vi "ConfigDlg.vi"(8 "error in (no error)":errorcluster, 11 "NiPxi6733 in":refnum<class "NiPxi6733.lvclass">) -> (0 "error out":errorcluster, 2 "Changed":bool, 3 "NiPxi6733 out":refnum<class "NiPxi6733.lvclass">)   [LabVIEW 2014, in "FgenPlugins.lvlib" / "NiPxi6733.lvclass"]
uses:
  NiPxi6733.lvclass
  TypeDefs/Channels.ctl
  TypeDefs/Channel.ctl
  TypeDefs/RefClk.ctl
  TypeDefs/clTriggers.ctl
  TypeDefs/Trigger.ctl
  TypeDefs/TriggerType.ctl
  Typedefs/Timebase.ctl
  FgenPluginBaseClass/FgenPluginsBase.lvclass/FgenPluginsBase.ctl
  NiPxi6733.lvclass/NiPxi6733.ctl
  <userlib>/NIST/BaseClasses/BasePlugin_class/BasePlugin.lvclass/BasePlugin.ctl
  <userlib>/NIST/BaseClasses/BasePlugin_class/Accessors/Read PluginIniFilePath.vi
  FgenPluginBaseClass/Accessors/Write reference clock source (Internal).vi
  Accessors/Write SampleRate.vi
  FgenPluginBaseClass/Accessors/Write Triggers.vi
  Accessors/Write Timebase.vi
  FgenPluginBaseClass/Accessors/Write Channels.vi
  FgenPluginBaseClass/Accessors/Read FunctionClass.vi
  Accessors/Read SampleRate.vi
  FgenPluginBaseClass/Accessors/Write FunctionClass.vi
  FgenPluginBaseClass/Accessors/Read Channels.vi
  FgenPluginBaseClass/Accessors/Read reference clock source (Internal).vi
  FgenPluginBaseClass/Read Triggers.vi
  Accessors/Read Timebase.vi
  MemberClasses/FunctionBaseClass/FunctionBase.lvclass
  <vilib>/Utility/config.llb/NI_LVConfig.lvlib
  FgenPlugins.lvlib
panel:
  in  "Timebase":T1={"source"="/PXI1Slot6/PXI_Trig1", "rate"=18000000.0}
  in  "Triggers":T2
  in  "SampleRate":dbl
  in  "btnDone":bool
  in  "btnCancel":bool
  in  "btnFuncConfig":bool
  in  "RefClk":T5 caption="reference clock source" items=["Internal"=0, "External"=1, "RTSI Clock"=101]
  in  "Channels":T6
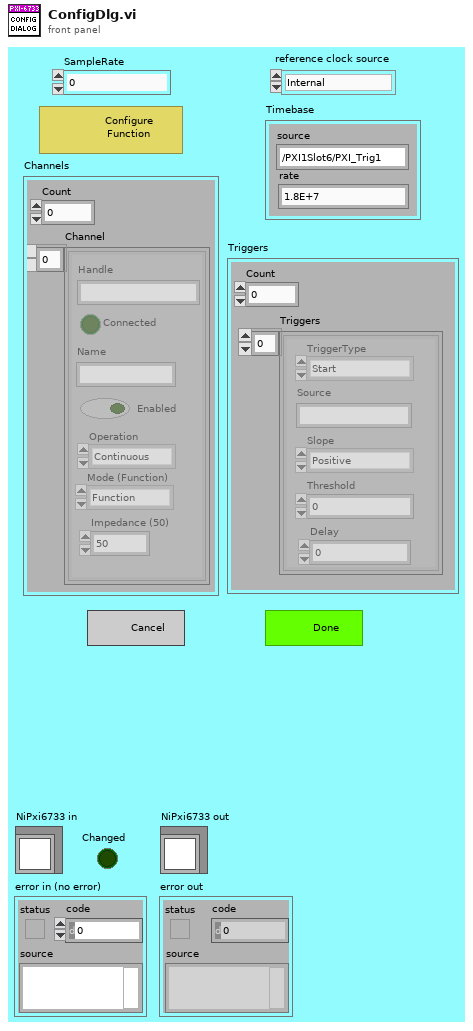
[diagram p1: front panel]
types:
  T1 = typedef "FgenPlugins.lvlib/NiPxi6733.lvclass/Timebase.ctl" = cluster{"source":string, "rate":dbl}
  T2 = typedef "FgenPlugins.lvlib/clTriggers.ctl" = cluster{"Count":i32, "Triggers":T3[]}
  T3 = typedef "FgenPlugins.lvlib/Trigger.ctl" = cluster{"Source":string, "Slope":enum16{"Positive", "Negative", "Either"}, "Threshold":dbl, "Delay":dbl, "TriggerType":T4}
  T4 = typedef "FgenPlugins.lvlib/TriggerType.ctl" = enum16{"None", "Start", "Stop", "Hold", "Resume", "Advance"}
  T5 = typedef "FgenPlugins.lvlib/RefClk.ctl" = i32
  T6 = typedef "FgenPlugins.lvlib/Channels.ctl" = cluster{"Count":u16, "Channel":T7[]}
  T7 = typedef "FgenPlugins.lvlib/Channel.ctl" = cluster{"Name":string, "Enabled":bool, "Operation":enum16{"Continuous", "Burst"}, "Impedance (50)":dbl, "Handle":string, "Connected":bool, "Mode (Function)":enum16{"Function", "Arbitrary", "Sequence"}}
  T8 = typedef "NI_LVConfig.lvlib/Config Data RefNum.ctl" = refnum<k1>
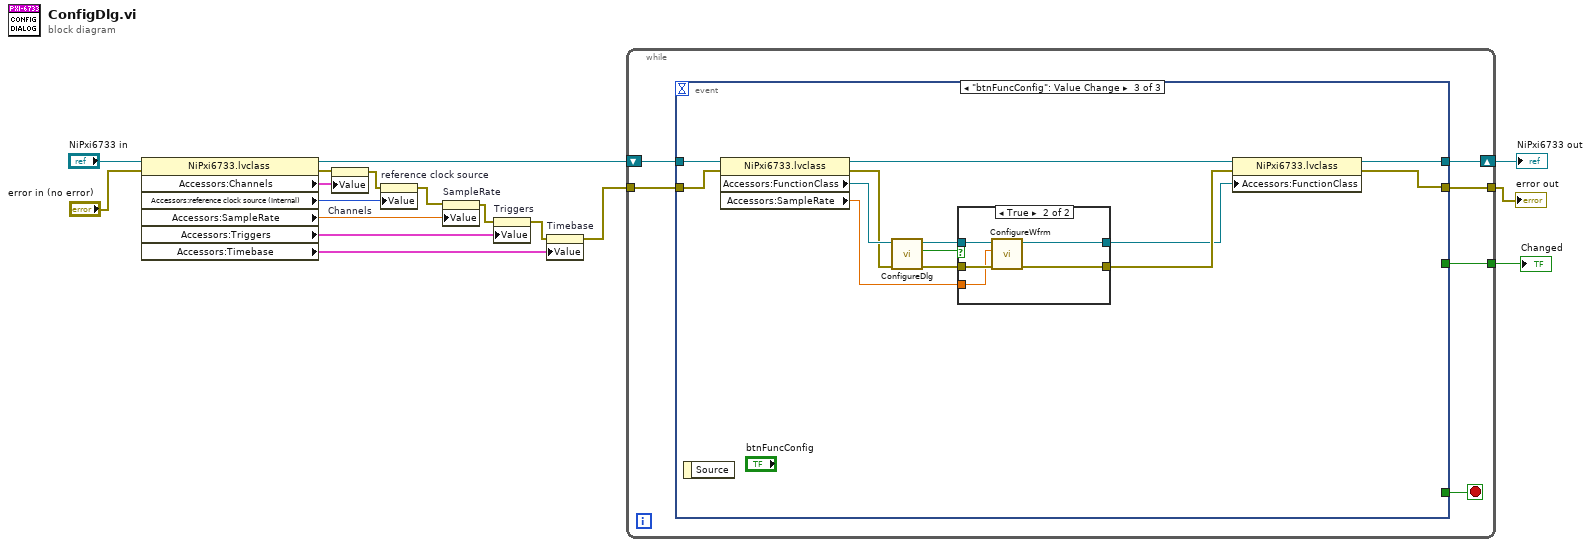
[diagram p0: block diagram]
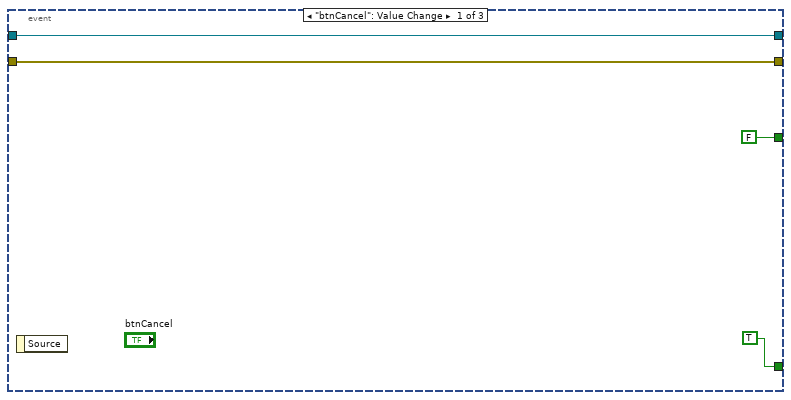
[diagram p2: hidden frame]
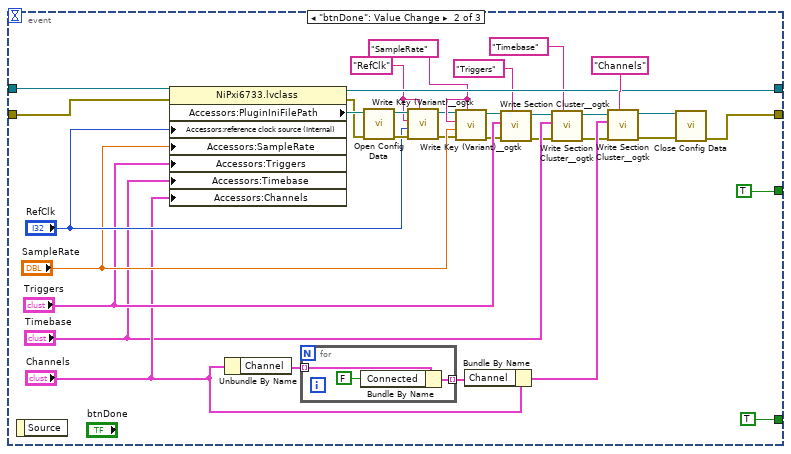
[diagram p3: hidden frame]
diagram:
  n1 = property class="NiPxi6733.lvclass"(reference="NiPxi6733 in", error in="error in (no error)") -> (reference out=w11:refnum<class "NiPxi6733.lvclass">, error out=w15:errorcluster, "Accessors:Channels"=w14:cluster{"Count":u16, "Channel":T7[]}, "Accessors:reference clock source (Internal)"=w13:i32, "Accessors:SampleRate"=w7:dbl, "Accessors:Triggers"=w5:T2, "Accessors:Timebase"=w3:T1)
  n2 = property on="Channels" class="Clust (strict)"(error in=w15, "Value"=w14) -> (error out=w12:errorcluster)  [unwired: 1 in, 1 out]
  n3 = property on="reference clock source" class="Ring (strict)"(error in=w12, "Value"=w13) -> (error out=w6:errorcluster)  [unwired: 1 in, 1 out]
  n4 = property on="SampleRate" class="DigNum (strict)"(error in=w6, "Value"=w7) -> (error out=w4:errorcluster)  [unwired: 1 in, 1 out]
  n5 = property on="Triggers" class="Clust (strict)"(error in=w4, "Value"=w5) -> (error out=w2:errorcluster)  [unwired: 1 in, 1 out]
  n6 = property on="Timebase" class="Clust (strict)"(error in=w2, "Value"=w3) -> (error out=w1:errorcluster)  [unwired: 1 in, 1 out]
  n7 = while {
    tunnel: [w21] -> w9
    tunnel: [w19] -> w8
    shift-right: [w22] -> w10
    shift-left: w11 -> [w23]
    tunnel: w1 -> [w18]
    stop <- w20 stop-if-true
    n8 = event shown="[2] \"btnFuncConfig\": Value Change" {
      selector: _ -> [_ _ _]
      dyn-events: _ -> [_ _ _]
      timeout: _ -> [_ _ _]
      tunnel: w23 -> [w27 w60 w76]
      tunnel: [w27 w52 w73] -> w22
      tunnel: [w24 w51 w70] -> w21
      tunnel: [TRUE TRUE _] -> w20
      tunnel: [FALSE TRUE _] -> w19
      tunnel: w18 -> [w24 w48 w72]
      event "btnCancel": Value Change {
        n9 = event-data() -> ()  [unwired: 1 in, 1 out]
      }
      event "btnDone": Value Change {
        w49 = "SampleRate" ("section (optional)")
        w40 = "RefClk" ("section")
        n10 = event-data() -> ()  [unwired: 1 in, 1 out]
        n11 = property class="NiPxi6733.lvclass"(reference=w60, error in=w48, "Accessors:reference clock source (Internal)"="RefClk", "Accessors:SampleRate"="SampleRate", "Accessors:Triggers"="Triggers", "Accessors:Timebase"="Timebase", "Accessors:Channels"="Channels") -> (reference out=w52:refnum<class "NiPxi6733.lvclass">, error out=w58:errorcluster, "Accessors:PluginIniFilePath"=w59:path)
        n12 = Unbundle By Name("Channels") -> ("Channel"=w46:T7[])
        n13 = for {
          tunnel: w46 -> [w63] mode=indexing
          tunnel: [w61] -> w45 mode=indexing
          n14 = Bundle By Name(cluster=w63, "Connected"=FALSE) -> (w61:T7)
        }
        n15 = call <vilib>:"Open Config Data.vi"("error in (no error)"=w58, "configuration file path"=w59) -> ("error out"=w57:errorcluster, "refnum"=w56:T8)  [unwired: 7 in, 1 out]
        n16 = call <userlib>:"Write Key (Variant)__ogtk.vi"("section"=w40, "error in (no error)"=w57, "key-value"="RefClk", "key (optional)"=w40, "refnum"=w56) -> ("error out"=w31:errorcluster, "refnum out"=w35:T8)  [unwired: 5 in]
        n17 = call <userlib>:"Write Key (Variant)__ogtk.vi"("section"=w49, "error in (no error)"=w31, "key-value"="SampleRate", "key (optional)"=w49, "refnum"=w35) -> ("error out"=w30:errorcluster, "refnum out"=w34:T8)  [unwired: 5 in]
        n18 = Bundle By Name(cluster="Channels", "Channel"=w45) -> (w44:T6)
        n19 = call <userlib>:"Write Section Cluster__ogtk.vi"("section (optional)"="Triggers", "error in (no error)"=w30, "Section Formatted Cluster"="Triggers", "refnum"=w34) -> ("error out"=w29:errorcluster, "dup refnum"=w33:T8)  [unwired: 6 in]
        n20 = call <userlib>:"Write Section Cluster__ogtk.vi"("section (optional)"="Timebase", "error in (no error)"=w29, "Section Formatted Cluster"="Timebase", "refnum"=w33) -> ("error out"=w28:errorcluster, "dup refnum"=w32:T8)  [unwired: 6 in]
        n21 = call <userlib>:"Write Section Cluster__ogtk.vi"("section (optional)"="Channels", "error in (no error)"=w28, "Section Formatted Cluster"=w44, "refnum"=w32) -> ("error out"=w42:errorcluster, "dup refnum"=w43:T8)  [unwired: 6 in]
        n22 = call <vilib>:"Close Config Data.vi"("error in (no error)"=w42, "refnum"=w43) -> ("error out"=w51:errorcluster)  [unwired: 8 in, 1 out]
      }
      event "btnFuncConfig": Value Change {
        n23 = event-data() -> ()  [unwired: 1 in, 1 out]
        n24 = property class="NiPxi6733.lvclass"(reference=w76, error in=w72) -> (reference out=w74:refnum<class "NiPxi6733.lvclass">, error out=w71:errorcluster, "Accessors:FunctionClass"=w75:refnum<class "FunctionBase.lvclass">, "Accessors:SampleRate"=w64:dbl)
        n25 = call-dynamic "ConfigureDlg.vi"("error in (no error)"=w71, "FunctionBase in"=w75) -> ("error out"=w68:errorcluster, "Changed"=w65:bool, "FunctionBase out"=w69:refnum<class "FunctionBase.lvclass">)  [unwired: 7 in]
        n26 = case shown="True" w65 {
          tunnel: w69 -> [w78 w83]
          tunnel: w68 -> [w77 w82]
          tunnel: [w77 w81] -> w67
          tunnel: [w78 w80] -> w66
          tunnel: w64 -> [_ w79]
          frame False {
          }
          frame True {
            n27 = call-dynamic "ConfigureWfrm.vi"("error in (no error)"=w82, "SampleRate"=w79, "FunctionBase in"=w83) -> ("error out"=w81:errorcluster, "FunctionBase out"=w80:refnum<class "FunctionBase.lvclass">)  [unwired: 7 in]
          }
        }
        n28 = property class="NiPxi6733.lvclass"(reference=w74, error in=w67, "Accessors:FunctionClass"=w66) -> (reference out=w73:refnum<class "NiPxi6733.lvclass">, error out=w70:errorcluster)
      }
    }
  }
  "error out" <- w9
  "NiPxi6733 out" <- w10
  "Changed" <- w8
